vi "IAmGLF-DeleteDVR.vi"(8 "error in (no error)":errorcluster, 11 "IAmGLF in":refnum<class "IAmGLF.lvclass">) -> (0 "error out":errorcluster, 3 "IAmGLF out":refnum<class "IAmGLF.lvclass">)   [LabVIEW 2024, in "GLF.lvlib" / "IAmGLF.lvclass"]
doc: "<B>Summary</B>\nTo delete the class DVR from standalone process."
uses:
  IAmGLF.lvclass
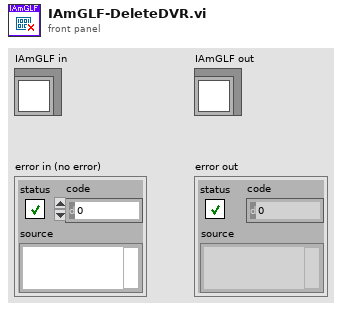
[diagram p1: front panel]
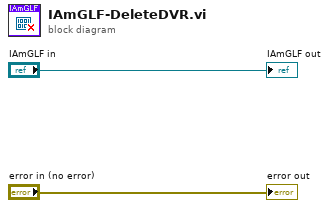
[diagram p0: block diagram]
diagram:
  "error out" <- "error in (no error)"
  "IAmGLF out" <- "IAmGLF in"
